vi "LAS-CTS_NDFilterRepeatabilityByStep.vi"() -> ()   [LabVIEW 2024]
uses:
  <vilib>/httpClient/LabVIEWHTTPClient.lvlib
  <vilib>/Analysis/NI_AALBase.lvlib
panel:
  out "Filename":path
  in  "File #":i32 format="%03d"
  in  "base filename":string
  in  "Target ID":string
  out "Laser Energy Chart":dbl(graph)
  out "Average Laser Energy (uJ)":dbl format="%.3g"
  out "ND Filter Position":i32
  in  "Filepath":path
  in  "# of Repetitions":i32
  in  "ND Filter Position":i32
  in  "ND Filter":refnum<visa-resource-name>
  in  "# of Pulses":i32
  out "# of measurements":i32
  out "Laser Energy (uJ)":dbl
  in  "Energy Meter":refnum<visa-resource-name>
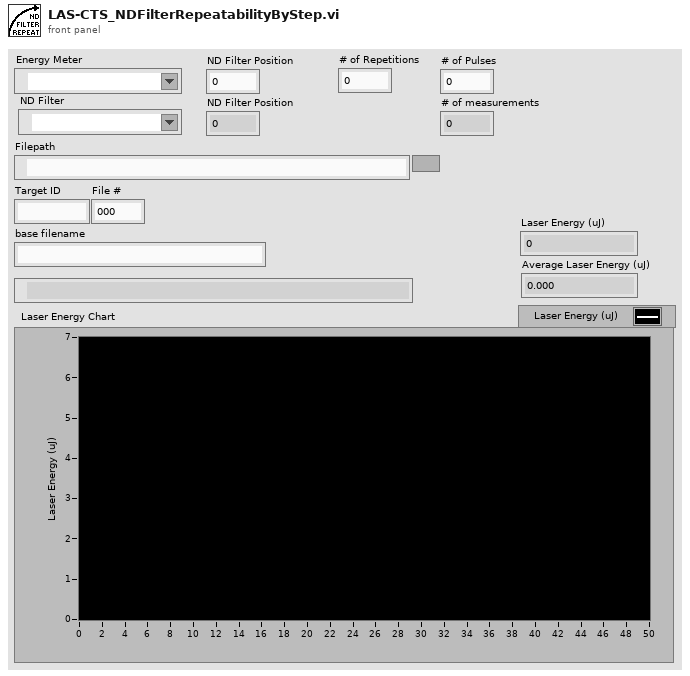
[diagram p1: front panel]
types:
  T1 = enum16{"open", "replace", "create", "open or create", "replace or create", "replace or create with confirmation"}
  T2 = typedef "LabVIEWHTTPClient.lvlib/ClientHandle.ctl" = refnum<k1>
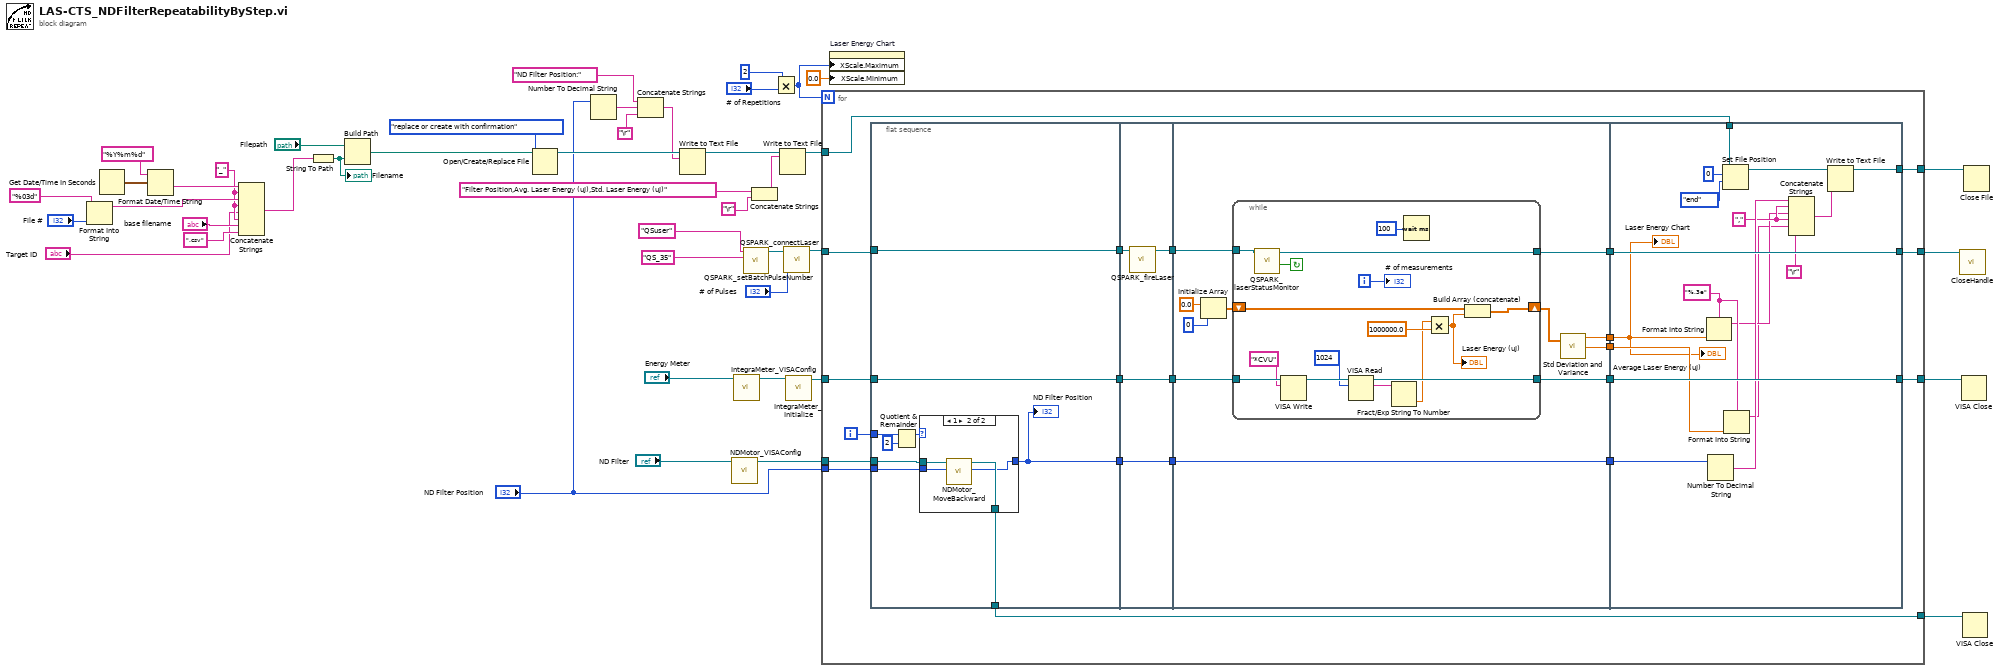
[diagram p0: block diagram]
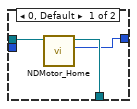
[diagram p2: hidden frame]
diagram:
  w7 = "_" ("string")
  n1 = Format Into String(format string="%03d", "File #") -> (resulting string=w8:string)  [unwired: 2 in, 1 out]
  n2 = Get Date/Time In Seconds() -> (seconds since 1Jan1904=w13:timestamp)
  n3 = Format Date/Time String(time format string (%c)="%Y%m%d", seconds (now)=w13) -> (date/time string=w11:string)  [unwired: 1 in]
  n4 = Concatenate Strings(w11, w7, w8, w7, "Target ID", w7, "base filename", ".csv" ("string")) -> (w14:string)
  n5 = String To Path(string=w14) -> (path=w4:path)
  "Filename" <- w4
  n6 = Build Path(base path="Filepath", name or relative path=w4) -> (appended path=w2:path)
  n7 = Open/Create/Replace File(file path (use dialog)=w2, operation (0:open)=T1."replace or create with confirmation") -> (refnum out=w20:refnum<file>)  [unwired: 4 in, 2 out]
  n8 = Number To Decimal String(number="ND Filter Position") -> (decimal integer string=w17:string)  [unwired: 1 in]
  n9 = Concatenate Strings("ND Filter Position:", w17, "\r") -> (w15:string)
  n10 = Write to Text File(file (use dialog)=w20, text=w15) -> (refnum out=w21:refnum<file>)  [unwired: 2 in, 2 out]
  n11 = call "NDMotor_VISAConfig.vi"("VISA resource name"="ND Filter") -> ("reference out"=w25:refnum<visa-resource-name>)  [unwired: 9 in, 1 out]
  n12 = call "IntegraMeter_VISAConfig.vi"("VISA resource name"="Energy Meter") -> ("reference out"=w44:refnum<visa-resource-name>)  [unwired: 9 in, 1 out]
  n13 = call "QSPARK_connectLaser.vi"("password"="QS_35", "username"="QSuser") -> ("client handle out"=w37:T2)  [unwired: 9 in]
  n14 = Concatenate Strings("Filter Position,Avg. Laser Energy (uJ),Std. Laser Energy (uJ)" ("text"), "\r") -> (w31:string)
  n15 = Multiply(x=2, y="# of Repetitions") -> (x*y=w22:i32)
  n16 = Write to Text File(file (use dialog)=w21, text=w31) -> (refnum out=w30:refnum<file>)  [unwired: 2 in, 2 out]
  n17 = call "QSPARK_setBatchPulseNumber.vi"("Number of Pulses"="# of Pulses", "client handle"=w37) -> ("client handle out"=w40:T2)  [unwired: 9 in]
  n18 = call "IntegraMeter_Initialize.vi"("VISA resource name"=w44) -> ("VISA resource name out"=w42:refnum<visa-resource-name>)  [unwired: 9 in, 1 out]
  n19 = for {
    N: w22 -> [_]
    tunnel: "ND Filter Position" -> [w50]
    tunnel: w30 -> [w57]
    tunnel: w40 -> [w61]
    tunnel: [w60] -> w38
    tunnel: w42 -> [w63]
    tunnel: [w62] -> w41
    tunnel: [w56] -> w29
    tunnel: [w46] -> w27
    tunnel: w25 -> [w51]
    i -> [w45]
    n20 = flat-sequence {
      tunnel: w63 -> [w73]
      tunnel: w61 -> [w74]
      tunnel: [w74] -> w53
      tunnel: [w73] -> w52
      tunnel: w51 -> [w72]
      tunnel: w45 -> [w71]
      tunnel: w50 -> [w69]
      tunnel: [w66] -> w47
      tunnel: [w68] -> w46
      tunnel: [w85] -> w65
      tunnel: [w83] -> w64
      tunnel: w53 -> [w84]
      tunnel: w52 -> [w85]
      tunnel: [w82] -> w48
      tunnel: w47 -> [w82]
      tunnel: w65 -> [w96]
      tunnel: w64 -> [w94]
      tunnel: [w95] -> w59
      tunnel: [w93] -> w58
      tunnel: [w89] -> w55
      tunnel: [w88] -> w54
      tunnel: [w86] -> w49
      tunnel: w48 -> [w86]
      tunnel: w59 -> [w129]
      tunnel: w58 -> [w128]
      tunnel: w57 -> [w125]
      tunnel: w55 -> [w118]
      tunnel: w54 -> [w120]
      tunnel: [w129] -> w62
      tunnel: [w128] -> w60
      tunnel: [w123] -> w56
      tunnel: w49 -> [w117]
      frame #0 {
        n21 = Quotient & Remainder(x=w71, y=2) -> (x-y*floor(x/y)=w67:i32)  [unwired: 1 out]
        n22 = case shown="1" w67 {
          tunnel: w72 -> [w77 w81]
          tunnel: w69 -> [_ w80]
          tunnel: [w75 w78] -> w66
          tunnel: [w76 w79] -> w68
          frame 0, Default {
            n23 = call "NDMotor_Home.vi"("VISA resource name"=w77) -> ("home offset steps"=w75:i32, "VISA resource name out"=w76:refnum<visa-resource-name>)  [unwired: 7 in, 2 out]
          }
          frame 1 {
            n24 = call "NDMotor_MoveBackward.vi"("Steps"=w80, "VISA resource name"=w81) -> ("steps"=w78:i32, "VISA resource name out"=w79:refnum<visa-resource-name>)  [unwired: 6 in, 2 out]
          }
        }
        "ND Filter Position" <- w66
      }
      frame #1 {
        n25 = call "QSPARK_fireLaser.vi"("client handle"=w84) -> ("client handle out"=w83:T2)  [unwired: 10 in]
      }
      frame #2 {
        n26 = Initialize Array(0.0 ("element"), 0 ("dimension size")) -> (w87:dbl[])
        n27 = while {
          tunnel: w96 -> [w112]
          tunnel: [w110] -> w95
          tunnel: w94 -> [w105]
          tunnel: [w104] -> w93
          shift-right: [w101] -> w90
          shift-left: w87 -> [w102]
          i -> [w106]
          stop <- w103 continue-if-true
          n28 = call "QSPARK_laserStatusMonitor.vi"("client handle"=w105) -> ("laser on?"=w103:bool, "client handle out"=w104:T2)  [unwired: 8 in, 1 out]
          n29 = VISA Write(VISA resource name=w112, write buffer="*CVU") -> (VISA resource name out=w111:refnum<visa-resource-name>)  [unwired: 1 in, 2 out]
          n30 = VISA Read(VISA resource name=w111, byte count=u32 1024) -> (VISA resource name out=w110:refnum<visa-resource-name>, read buffer=w107:string)  [unwired: 1 in, 2 out]
          n31 = Fract/Exp String To Number(string=w107) -> (number=w98:dbl)  [unwired: 3 in, 1 out]
          n32 = Wait (ms)(milliseconds to wait=u32 100 ("millisecond multiple")) -> ()  [unwired: 1 out]
          n33 = Multiply(x=w98, y=1000000.0) -> (x*y=w97:dbl)
          "Laser Energy (uJ)" <- w97
          n34 = Build Array (concatenate)(w102, w97) -> (w101:dbl[])
          "# of measurements" <- w106
        }
        n35 = call <vilib>:"Std Deviation and Variance.vi"("X"=w90) -> ("mean"=w89:dbl, "standard deviation"=w88:dbl)  [unwired: 1 in, 1 out]
      }
      frame #3 {
        w116 = "," ("string")
        w121 = "%.3e" ("format string")
        n36 = Format Into String(format string=w121, w118) -> (resulting string=w115:string)  [unwired: 2 in, 1 out]
        n37 = Number To Decimal String(number=w117) -> (decimal integer string=w119:string)  [unwired: 1 in]
        n38 = Set File Position(offset (in bytes) (0)=i64 0, refnum=w125, from (0:start)=enum16{"start", "end", "current"}."end") -> (refnum out=w124:refnum<file>)  [unwired: 1 in, 1 out]
        n39 = Format Into String(format string=w121, w120) -> (resulting string=w114:string)  [unwired: 2 in, 1 out]
        n40 = Concatenate Strings(w119, w116, w115, w116, w114, "\r") -> (w122:string)
        n41 = Write to Text File(file (use dialog)=w124, text=w122) -> (refnum out=w123:refnum<file>)  [unwired: 2 in, 2 out]
        "Average Laser Energy (uJ)" <- w118
        "Laser Energy Chart" <- w118
      }
    }
  }
  n42 = property on="Laser Energy Chart" class="WFChart (strict)"("XScale.Maximum"=w22, "XScale.Minimum"=0.0 ("X Scale.Range:Minimum")) -> ()  [unwired: 2 in, 2 out]
  n43 = call <vilib>:"CloseHandle.vi"("client handle"=w38) -> ()  [unwired: 14 in, 1 out]
  n44 = VISA Close(VISA resource name=w41) -> ()  [unwired: 1 in, 1 out]
  n45 = VISA Close(VISA resource name=w27) -> ()  [unwired: 1 in, 1 out]
  n46 = Close File(refnum=w29) -> ()  [unwired: 1 in, 2 out]
